vi "data load(SubVI).vi"(11 "file path":path caption="文件路径 （空时为对话框）") -> (1 "数据起始行":i32, 2 "项名":string[](array[string]))   [LabVIEW 2019, in "SubVI.lvlib"]
uses:
  SubVI.lvlib
  <vilib>/Utility/file.llb/Read Delimited Spreadsheet (string).vi
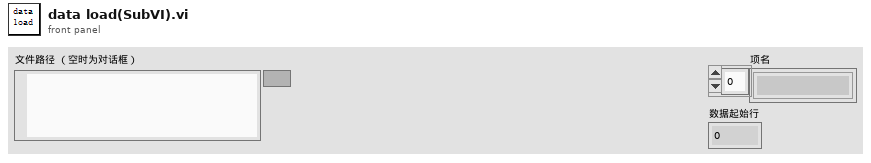
[diagram p1: front panel]
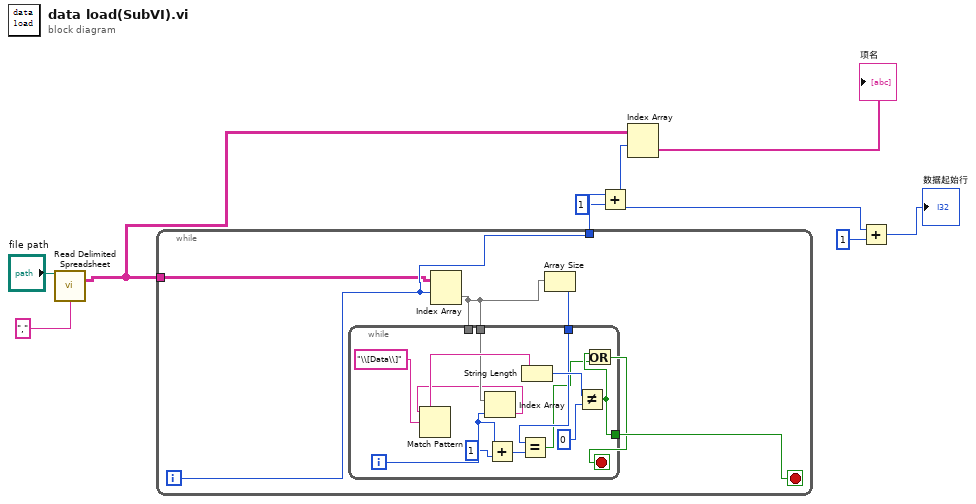
[diagram p0: block diagram]
diagram:
  n1 = call-poly <vilib>:"Read Delimited Spreadsheet.vi"("file path (dialog if empty)"="file path", "delimiter (\\t)"="," ("delimiter (\\t)")) -> ("all rows"=w8:string[][])  [unwired: 8 in, 5 out]
  n2 = while {
    tunnel: [w11] -> w7
    tunnel: w8 -> [w10]
    i -> [w11]
    stop <- w14 stop-if-true
    n3 = Index Array(array=w10, index (row)=w11) -> (element=w13:string[])  [unwired: 1 in]
    n4 = Array Size(array=w13) -> (size(s)=w12:i32)
    n5 = while {
      tunnel: [w18] -> w14
      tunnel: w13 -> [_]
      tunnel: w13 -> [w23]
      tunnel: w12 -> [w22]
      i -> [w21]
      stop <- w16 stop-if-true
      n6 = Index Array(array=w23, index=w21) -> (element=w15:string)
      n7 = Match Pattern(string=w15, regular expression="\\[Data\\]" ("正则表达式")) -> (match substring=w26:string)  [unwired: 1 in, 3 out]
      n8 = Add(x=w21, y=1) -> (x+y=w19:i32)
      n9 = Equal?(x=w22, y=w19) -> (x = y?=w17:bool)
      n10 = String Length(string=w26) -> (length=w25:i32)
      n11 = Not Equal?(x=w25, y=0) -> (x != y?=w18:bool)
      n12 = Or(x=w18, y=w17) -> (x .or. y?=w16:bool)
    }
  }
  n13 = Add(x=w7, y=1) -> (x+y=w4:i32)
  n14 = Index Array(array=w8, index (row)=w4) -> (element=→"项名":string[])  [unwired: 1 in]
  n15 = Add(x=w4, y=1) -> (x+y=→"数据起始行":i32)
